vi "Tags.ChangePath.vi"(8 "error in (no error)":errorcluster, 10 "Name":string, 11 "Section Ref in":T1 format="%.0x") -> (0 "error out":errorcluster)   [LabVIEW 2019, in "OPC UA Client Addon System Explorer.lvlib"]
uses:
  OPC UA Client Addon System Explorer.lvlib
  <vilib>/NI VeriStand/Custom Device Tools/Custom Device Utility Library/Custom Device Utility Library.lvlib
  <vilib>/NI VeriStand/Custom Device Tools/Custom Device Utility Library/NI VeriStand - Search for All Items by GUID.vi
  Addon Shared/SubVIs/Constants.vi
  Addon Shared/OPC UA Client Addon Shared.lvlib
  <vilib>/NI VeriStand/Custom Device API/Custom Device API.lvlib
  <vilib>/NI VeriStand/Custom Device API/Set Item Property (String).vi
  <vilib>/NI VeriStand/Custom Device API/Get Item Property (String).vi
  <vilib>/NI VeriStand/Custom Device API/Custom Device Item Ref.ctl
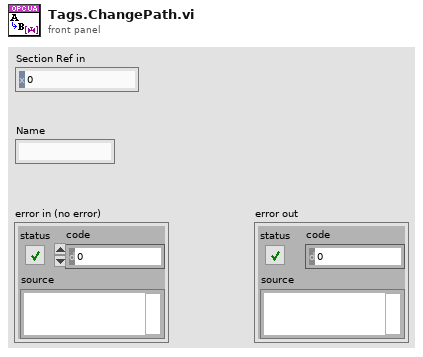
[diagram p1: front panel]
types:
  T1 = typedef "Custom Device API.lvlib/Custom Device Item Ref.ctl" = u64
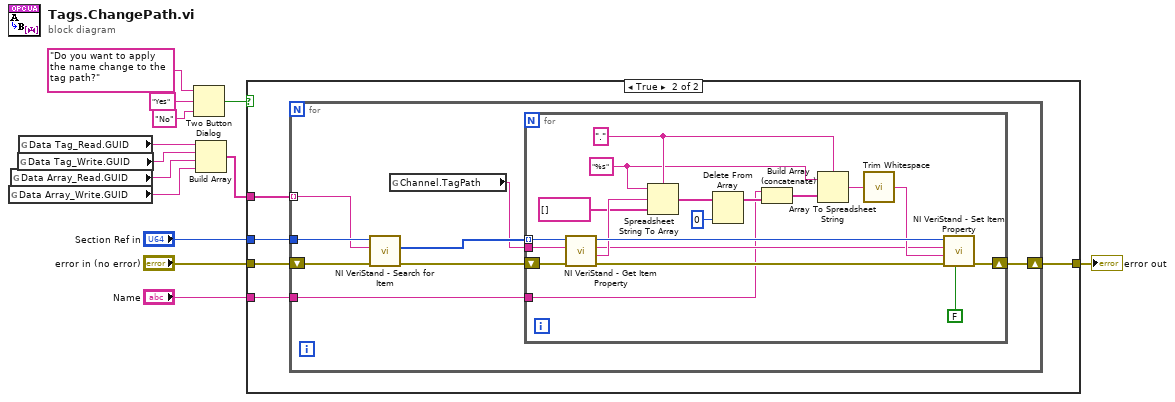
[diagram p0: block diagram]
diagram:
  n1 = global read "Constants.vi" "Data Array_Write.GUID"() -> (w1:string)
  n2 = global read "Constants.vi" "Data Array_Read.GUID"() -> (w2:string)
  n3 = global read "Constants.vi" "Data Tag_Write.GUID"() -> (w5:string)
  n4 = global read "Constants.vi" "Data Tag_Read.GUID"() -> (w6:string)
  n5 = Two Button Dialog(message="Do you want to apply the name change to the tag path?", 1:"No" ("F button name (\"Cancel\")"), 2:"Yes" ("T button name (\"OK\")")) -> (T button?=w11:bool)
  n6 = Build Array(w6, w5, w2, w1) -> (w4:string[])
  n7 = case shown="True" w11 {
    tunnel: "error in (no error)" -> [w14 w19]
    tunnel: [w14 w18] -> w13
    tunnel: "Section Ref in" -> [_ w17]
    tunnel: w4 -> [_ w16]
    tunnel: "Name" -> [_ w15]
    frame False {
    }
    frame True {
      n8 = for {
        shift-right: [w22] -> w18
        shift-left: w19 -> [w27]
        tunnel: w17 -> [w26]
        tunnel: w16 -> [w25] mode=indexing
        tunnel: w15 -> [w20]
        n9 = call-poly <vilib>:"NI VeriStand - Search for Item.vi"("error in"=w27, "Item GUID"=w25, "Section Ref in"=w26) -> ("error out"=w23:errorcluster, "Item Refs"=w24:T1[])  [unwired: 5 in, 2 out]
        n10 = global read "Constants.vi" "Channel.TagPath"() -> (w21:string)
        n11 = for {
          tunnel: w24 -> [w45] mode=indexing
          shift-right: [w42] -> w22
          shift-left: w23 -> [w44]
          tunnel: w21 -> [w29]
          tunnel: w20 -> [w28]
          w37 = "%s" ("format string")
          w38 = "." ("delimiter (Tab)")
          n12 = call-poly <vilib>:"NI VeriStand - Get Item Property.vi"("error in (no error)"=w44, "Property Name"=w29, "Item Ref in"=w45) -> ("error out"=w43:errorcluster, "Value"=w39:string, "Item Ref out"=w40:T1)  [unwired: 5 in, 1 out]
          n13 = Spreadsheet String To Array(delimiter (Tab)=w38, format string=w37, spreadsheet string=w39, array type (2D Dbl)=string[] []) -> (array=w35:string[])
          n14 = Delete From Array(array=w35, index=0) -> (array with subset deleted=w33:string[])  [unwired: 1 in, 1 out]
          n15 = Build Array (concatenate)(w28, w33) -> (w32:string[])
          n16 = Array To Spreadsheet String(delimiter (Tab)=w38, array=w32, 3:w37) -> (spreadsheet string=w31:string)
          n17 = call <vilib>:"Trim Whitespace.vi"("string"=w31) -> ("trimmed string"=w30:string)  [unwired: 1 in]
          n18 = call-poly <vilib>:"NI VeriStand - Set Item Property.vi"("Binary String (T)"=FALSE, "error in (no error)"=w43, "Value"=w30, "Property Name"=w29, "Item Ref in"=w40) -> ("error out"=w42:errorcluster)  [unwired: 4 in, 2 out]
        }
      }
    }
  }
  "error out" <- w13
